vi "Global-1.vi"() -> ()   [LabVIEW 2014]
panel:
  out "opening width":dbl=4.0
  out "Score":dbl
  in  "score points":dbl[](array[numeric])
  out "H-speed":dbl
  in  "yu":dbl[](array[numeric])
  in  "yl":dbl[](array[numeric])
  in  "x":dbl[](array[numeric])
  out "Up index":i32
  # "first point is AP1 \nlast point is AP2"
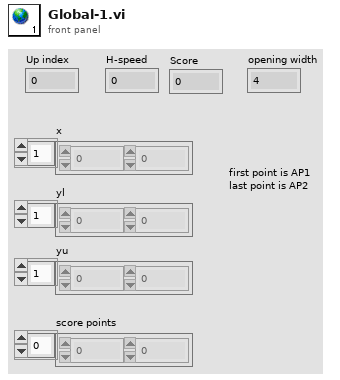
[diagram p1: front panel]
diagram:
